vi "setSetpoint.vi"(0 "SingleCylinderActuator in":refnum<class "SingleCylinderActuator.lvclass">, 5 "Flow Control Setpoint":dbl[unit], 7 "Pressure Servo Valve 1 Setpoint":dbl[unit], 9 "Pressure Servo Valve 2 Setpoint":dbl[unit], 11 "error in (no error)":errorcluster) -> (4 "SingleCylinderActuator out":refnum<class "SingleCylinderActuator.lvclass">, 15 "error out":errorcluster)   [LabVIEW 2015, in "SingleCylinderActuator.lvclass"]
uses:
  SingleCylinderActuator.lvclass
  ActuatorCylinder/IActuatorCylinder/IActuatorCylinder.lvclass
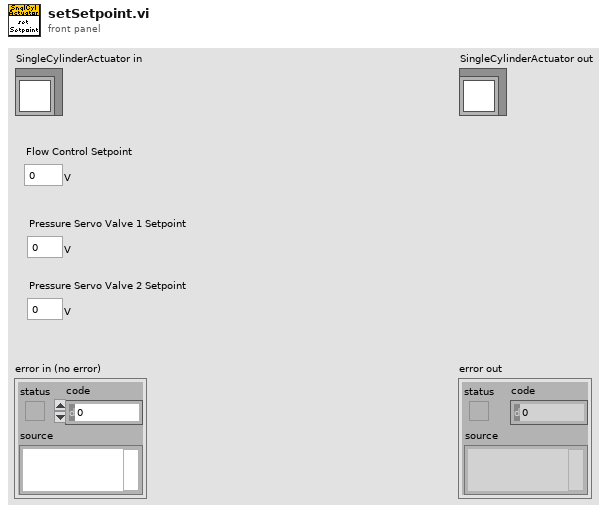
[diagram p1: front panel]
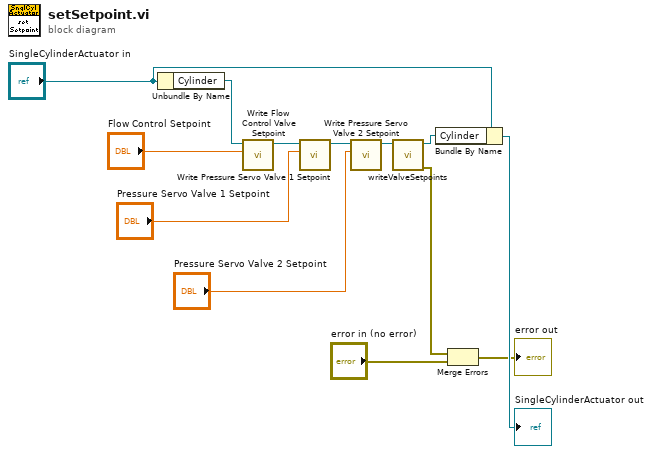
[diagram p0: block diagram]
diagram:
  n1 = Unbundle By Name("SingleCylinderActuator in") -> ("Cylinder"=w3:refnum<class "IActuatorCylinder.lvclass">)
  n2 = call-dynamic "Write Flow Control Valve Setpoint.vi"("Flow Control Valve Setpoint"="Flow Control Setpoint", "IActuatorCylinder in"=w3) -> ("IActuatorCylinder out"=w2:refnum<class "IActuatorCylinder.lvclass">)  [unwired: 9 in]
  n3 = call-dynamic "Write Pressure Servo Valve 1 Setpoint.vi"("Pressure Servo Valve 1 Setpoint"="Pressure Servo Valve 1 Setpoint", "IActuatorCylinder in"=w2) -> ("IActuatorCylinder out"=w1:refnum<class "IActuatorCylinder.lvclass">)  [unwired: 9 in]
  n4 = call-dynamic "Write Pressure Servo Valve 2 Setpoint.vi"("Pressure Servo Valve 2 Setpoint"="Pressure Servo Valve 2 Setpoint", "IActuatorCylinder in"=w1) -> ("IActuatorCylinder out"=w5:refnum<class "IActuatorCylinder.lvclass">)  [unwired: 9 in]
  n5 = call-dynamic "writeValveSetpoints.vi"("IActuatorCylinder in"=w5) -> ("error out"=w9:errorcluster, "IActuatorCylinder out"=w6:refnum<class "IActuatorCylinder.lvclass">)  [unwired: 9 in]
  n6 = Bundle By Name(cluster="SingleCylinderActuator in", "Cylinder"=w6) -> (→"SingleCylinderActuator out":refnum<class "SingleCylinderActuator.lvclass">)
  n7 = Merge Errors(w9, "error in (no error)") -> (→"error out":errorcluster)
